vi "Test Get Failed Items Include Broken.vi"(8 "error in (no error)":errorcluster, 11 "Result Model Result Recording Test in":refnum<class "Result Model Result Recording Test.lvclass">) -> (0 "error out":errorcluster, 3 "Result Model Result Recording Test out":refnum<class "Result Model Result Recording Test.lvclass">)   [LabVIEW 2020, in "Result Model Result Recording Test.lvclass"]
uses:
  Result Model Result Recording Test.lvclass
  source/Core/Result/Type.ctl
  source/Core/Result/Result.lvlib
  source/Core/Result/Status.ctl
  source/Core/Result/Result.ctl
  source/User Interface/Result Model/Result Model.lvclass
  ae2c71b8-32bb-49d1-8500-0119bfec74ff.vi
  source/User Interface/Result Model/Tree Item Filter.ctl
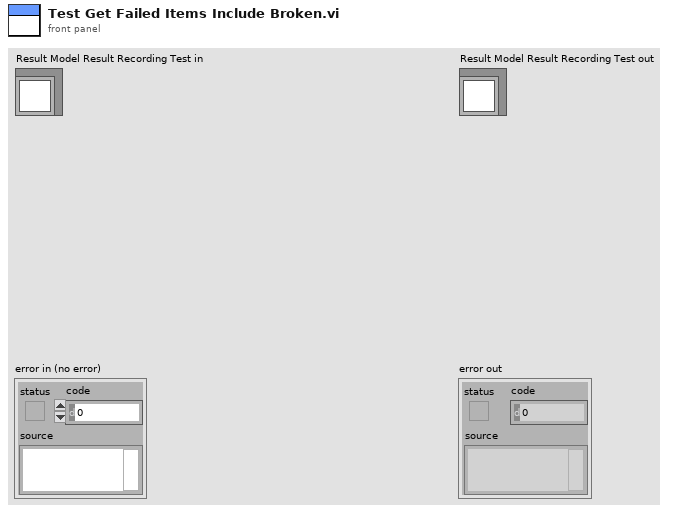
[diagram p1: front panel]
types:
  T1 = typedef "Result Model.lvclass/Tree Item Filter.ctl" = enum16{"All", "Only Fails", "Fails or else Not Executed"}
  T2 = typedef "Result.lvlib/Result.ctl" = cluster{"Name":string, "Description":string, "Status":T3, "Result Type":T4, "Execution Time":dbl, "Data":cluster{"Expected":variant, "Actual":variant, "Delta":variant}}
  T3 = typedef "Result.lvlib/Status.ctl" = enum16{"", "Passed", "Failed", "Error", "Skipped", "Setup Error", "Broken", "Teardown Error"}
  T4 = typedef "Result.lvlib/Type.ctl" = enum16{"Test Case", "Test Suite", "Test Run", "Pass", "Fail", "Skip", "Pass if", "Fail if", "Pass if Error", "Fail if Error", "Pass if Equal", "Fail if Equal"}
  T5 = cluster{"Left Cell String":string, "Child Text":string[], "Child Tag":string, "Item Indent":i32, "Child Only?":bool, "Glyph Index":i32}[]
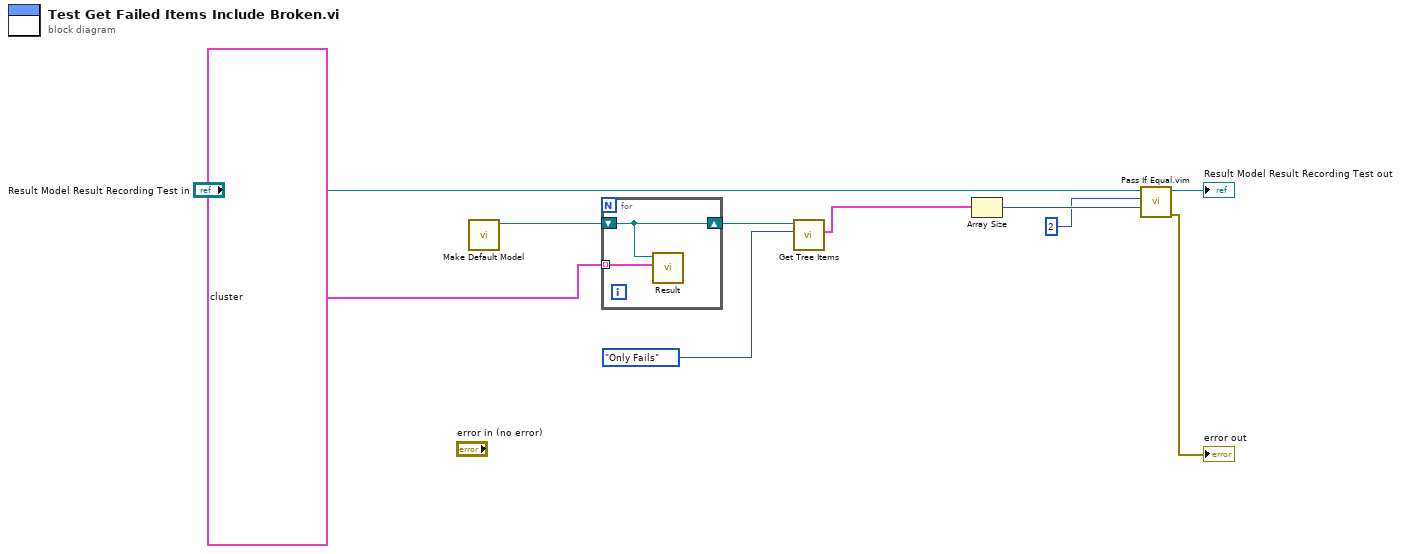
[diagram p0: block diagram]
diagram:
  n1 = call "Make Default Model.vi"() -> ("Result Model out"=w10:refnum<class "Result Model.lvclass">)  [unwired: 10 in, 1 out]
  n2 = for {
    tunnel: T2[] [{"Name"="Case.lvclass:Test Method.vi", "Description"="Failed:\nMessage", "Status"=enum."Broken", "Result Type"=enum."Test Case", "Execution Time"=0.107, "Data"={"Expected"=variant, "Actual"=variant, "Delta"=variant}}, {"Name"="Case.lvclass:Test Method2.vi", "Description"="", "Status"=enum."Passed", "Result Type"=enum."Test Case", "Execution Time"=0.0, "Data"={"Expected"=variant, "Actual"=variant, "Delta"=variant}}, {"Name"="Case.lvclass", "Description"="", "Status"=enum."Error", "Result Type"=enum."Test Suite", "Execution Time"=0.0, "Data"={"Expected"=variant, "Actual"=variant, "Delta"=variant}}] ("Results") -> [w12] mode=indexing
    shift-right: [w11] -> w8
    shift-left: w10 -> [w11]
    n3 = call-dynamic "Result.vi"("Results"=w12, "Result Model by Reference In"=w11) -> ()  [unwired: 9 in, 1 out]
  }
  n4 = call "Get Tree Items.vi"("Filter"=Tree_Item_Filter."Only Fails", "Result Model by Reference In"=w8) -> ("Tree Items"=w7:T5)  [unwired: 8 in, 1 out]
  n5 = Array Size(array=w7) -> (size(s)=w3:i32)
  n6 = call "Pass If Equal.vim"("Actual"=w3, "Expected"=2 ("size(s)"), "LUnit Test Case In"="Result Model Result Recording Test in") -> ("error out"=→"error out":errorcluster, "LUnit Test Case Out"=→"Result Model Result Recording Test out":refnum<class "Result Model Result Recording Test.lvclass">)  [unwired: 7 in]
